vi "Set Background Image.vi"(8 "error in (no error)":errorcluster, 10 "GUI ref in":refnum<vi>, 11 "Common GUI v3 in":refnum<class "Common GUI v3.lvclass">) -> (0 "error out":errorcluster, 2 "GUI ref out":refnum<vi>, 3 "Common GUI v3 out":refnum<class "Common GUI v3.lvclass">)   [LabVIEW 2026, in "TALOS.lvlib" / "Common GUI v3.lvlib" / "Common GUI v3.lvclass"]
uses:
  Common GUI v3.lvclass
  Ancestor/Ancestor/Ancestor.lvclass/Ancestor.ctl
  Support VIs/Generate Error.vi
  FGV/Error Memory/Get Error Description.vi
  Support VIs/Get PC name.vi
  Ancestor/Ancestor/Read ID.vi
  Support VIs/Get Class Name.vi
  <vilib>/Utility/error.llb/Clear Errors.vi
  FGV/Error Memory/Error Memory Core.vi
  <vilib>/AdvancedString/Delimited String to 1D String Array.vi
  <vilib>/AdvancedString/Delimited String to 1D String Array (string).vi
  Support VIs/Circus Root Path.vi
  FGV/Error Memory/Error Crt Lvl checker.vi
  FGV/Error Memory/Error Memory Core.vi/40c8088d-b597-4017-91af-faa98e00292e.vi
  FGV/Error Memory/Error Memory Core.vi/d4a3ab98-063c-4e44-b43d-fbdcfe6c2be2.vi
  Support VIs/Global Memory.vi
  <vilib>/Utility/LVClass/Get LV Class Name.vi
  Support VIs/Is in Packed Library.vi
  Support VIs/TALOS Root path.vi
  Support VIs/Read CSV worksheet.vi
  Support VIs/Global Constants.vi
  <vilib>/Utility/error.llb/General Error Handler.vi
  Support VIs/Error Log.vi
  Ancestor/Ancestor/Ancestor.lvclass
  <vilib>/Comparison/Equal/Equal Functor/Equal Functor.lvclass
  TALOS.lvlib
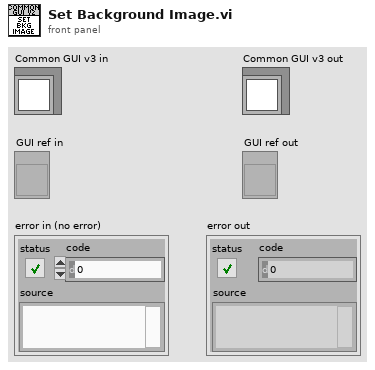
[diagram p1: front panel]
types:
  T1 = typedef "imagedata.ctl" = cluster{"image type":i32, "image depth":i32, "image":u8[], "mask":u8[], "colors":u32[], "Rectangle":cluster{"left":i16, "top":i16, "right":i16, "bottom":i16}}
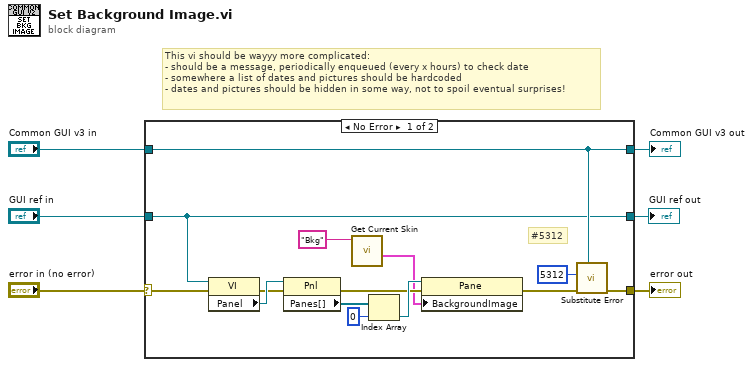
[diagram p0: block diagram]
diagram:
  # "This vi should be wayyy more complicated:\n- should be a message, periodically enqueued (every x hours) to check date\n- somewhere a list of dates and pictures should be hardcoded\n- dates and pictures should be hidden in some way, not to spoil eventual surprises!"
  n1 = case shown="No Error" "error in (no error)" {
    selector: "error in (no error)" -> [w9 w23]
    tunnel: "GUI ref in" -> [w10 w21]
    tunnel: [w20 w23] -> w5
    tunnel: "Common GUI v3 in" -> [w19 w22]
    tunnel: [w19 w22] -> w3
    tunnel: [w10 w21] -> w1
    frame No Error {
      # "#5312"
      n2 = property class="VI"(reference=w10, error in=w9) -> (error out=w12:errorcluster, "Panel"=w13:refnum<vi>)  [unwired: 1 out]
      n3 = property class="Pnl"(reference=w13, error in=w12) -> (error out=w11:errorcluster, "Panes[]"=w16:refnum<vi>[])  [unwired: 1 out]
      n4 = call "Get Current Skin.vi"("Object"="Bkg") -> ("image data"=w8:T1)  [unwired: 5 in, 2 out]
      n5 = Index Array(array=w16, index=0) -> (element=w14:refnum<vi>)
      n6 = property class="Pane"(reference=w14, error in=w11, "BackgroundImage"=w8) -> (error out=w17:errorcluster)  [unwired: 1 out]
      n7 = call "Substitute Error.vi"("LabVIEW Object"=w19, "error in (no error)"=w17, "Error Code"=5312) -> ("error out"=w20:errorcluster)  [unwired: 8 in]
    }
    frame Error {
    }
  }
  "error out" <- w5
  "Common GUI v3 out" <- w3
  "GUI ref out" <- w1
